vi "DsbScAM+_SubVI_.vi"(9 "Carrier Freq":dbl, 10 "sampling info":cluster{"Fs":dbl, "#s":dbl}, 11 "Modulation Freq":dbl) -> (3 "Waveform":waveform(dbl))   [LabVIEW 2011]
uses:
  <vilib>/measure/NI_MABase.lvlib
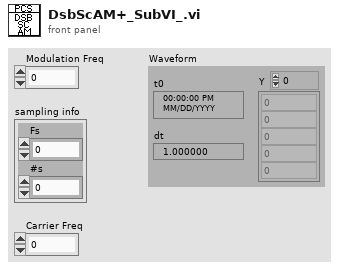
[diagram p1: front panel]
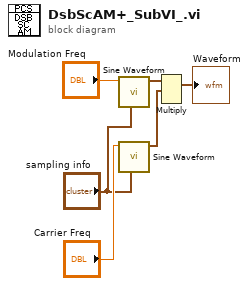
[diagram p0: block diagram]
diagram:
  n1 = call <vilib>:"Sine Waveform.vi"("sampling info"="sampling info", "frequency"="Modulation Freq") -> ("signal out"=w4:waveform(dbl))  [unwired: 8 in, 1 out]
  n2 = call <vilib>:"Sine Waveform.vi"("sampling info"="sampling info", "frequency"="Carrier Freq") -> ("signal out"=w5:waveform(dbl))  [unwired: 8 in, 1 out]
  n3 = Multiply(1:w5, 2:w4) -> (0:→"Waveform":waveform(dbl))  [unwired: 1 in, 1 out]
